vi "Config.File.Write.vi"(8 "error in":errorcluster, 11 "path":path) -> (0 "error out":errorcluster)   [LabVIEW 2016]
uses:
  Tma.lib/nlconfig.llb/fp2ini mode.ctl
  Global/ApplicationGlobal.vi
  Config.Global.vi
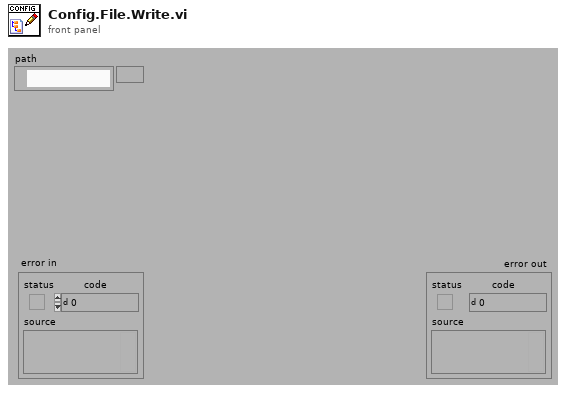
[diagram p1: front panel]
types:
  T1 = typedef "fp2ini mode.ctl" = enum16{"Read Controls", "Write Controls", "Write Indicators", "Read Indicators", "Write all", "Read all"}
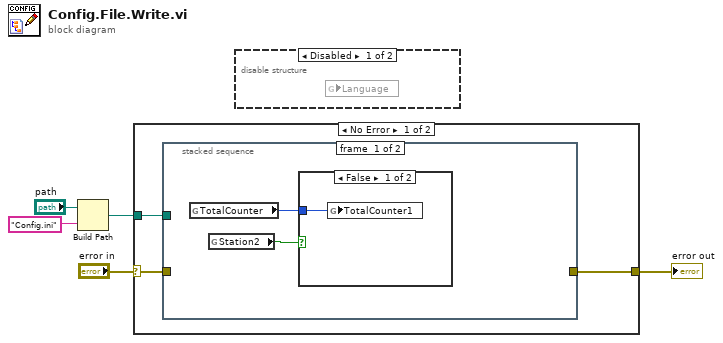
[diagram p0: block diagram]
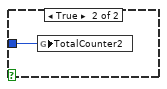
[diagram p3: hidden frame]
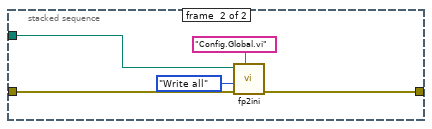
[diagram p4: hidden frame]
diagram:
  n1 = Build Path(base path="path", name or relative path="Config.ini") -> (appended path=w1:path)
  n2 = case shown="No Error" "error in" {
    selector: "error in" -> [w8 w18]
    tunnel: [w7 w18] -> w5
    tunnel: w1 -> [w6 _]
    frame No Error {
      n3 = stacked-sequence {
        tunnel: w8 -> [_ w15]
        tunnel: [_ w14] -> w7
        tunnel: w6 -> [_ w13]
        frame #0 {
          n4 = global read "ApplicationGlobal.vi" "TotalCounter"() -> (w10:u32)
          n5 = global read "ApplicationGlobal.vi" "Station2"() -> (w9:bool)
          n6 = case shown="False" w9 {
            tunnel: w10 -> [w11 w12]
            frame False {
              n7 = global write "Config.Global.vi" "TotalCounter1"(w11) -> ()
            }
            frame True {
              n8 = global write "Config.Global.vi" "TotalCounter2"(w12) -> ()
            }
          }
        }
        frame #1 {
          n9 = call "fp2ini.vi"("vi-name (caller if empty)"="Config.Global.vi", "error in"=w15, "mode"=fp2ini_mode."Write all", "ini-file path"=w13) -> ("error out"=w14:errorcluster)  [unwired: 7 in]
        }
      }
    }
    frame Error {
    }
  }
  "error out" <- w5
  n10 = disable-structure shown="Disabled" {
    frame Disabled {
      n11 = global read "Config.Global.vi" "Language"() -> ()  [unwired: 1 in]
    }
    frame Enabled {
    }
  }
